vi "eFGV - Data to Execute.vi"(6 "Action":T7, 8 "Error In":errorcluster, 10 "Data to Execute":T1={"Transaction Info"={"Transaction Number"="", "Order Number"="", "Quantity"=0, "Customer"=0, "Customer Description"="", "Project"="", "Sales Order"=0, "Material"="", "Material Description"="", "Rework"=FALSE, "NCR No."="", "Ref Order No."="", "Item No."=0, "BOM Rev."=0.0}, "Product Info"={"Product Category"="", "Procedure No./Ref."="", "Test System"="", "Test System Description"="", "Working Pressure"="", "Pressure Unit"="", "Rev."="", "PSL"=""}, "Misc - Additional Refs"=[], "Misc - Sensors"=[], "Misc - Tools"=[], "Acceptance Criteria Info"={"Max Start Hold Pressure"=0.0, "Enum.Max Start Hold Pressure"=enum."%", "Permitted Hold Pressure Drop"=0.0, "Enum.Permitted Hold Pressure Drop"=enum."%", "Pressure stabilize wait time"=10.0, "Enum.Pressure stabilize wait time"=enum."minutes"}, "Execution Info"={"Auto Set Marker"=FALSE, "Auto Stop Test"=FALSE}, "Results Info"={"ListBox.Output Set"="", "Output Set Description"=""}, "Notes"=""} {"Acceptance Criteria Info"."Pressure stabilize wait time" format="%#_13g"}) -> (0 "Error Out":errorcluster, 2 "Event - Data to Execute":refnum<user-event>)   [LabVIEW 2020]
uses:
  Control/State - eFGV.ctl
  Control/Data to Execute.ctl
  Control/Transaction Info.ctl
  Control/Product Info.ctl
  Control/Acceptance Criteria Info.ctl
  Control/Execution Info.ctl
  Control/Results Info.ctl
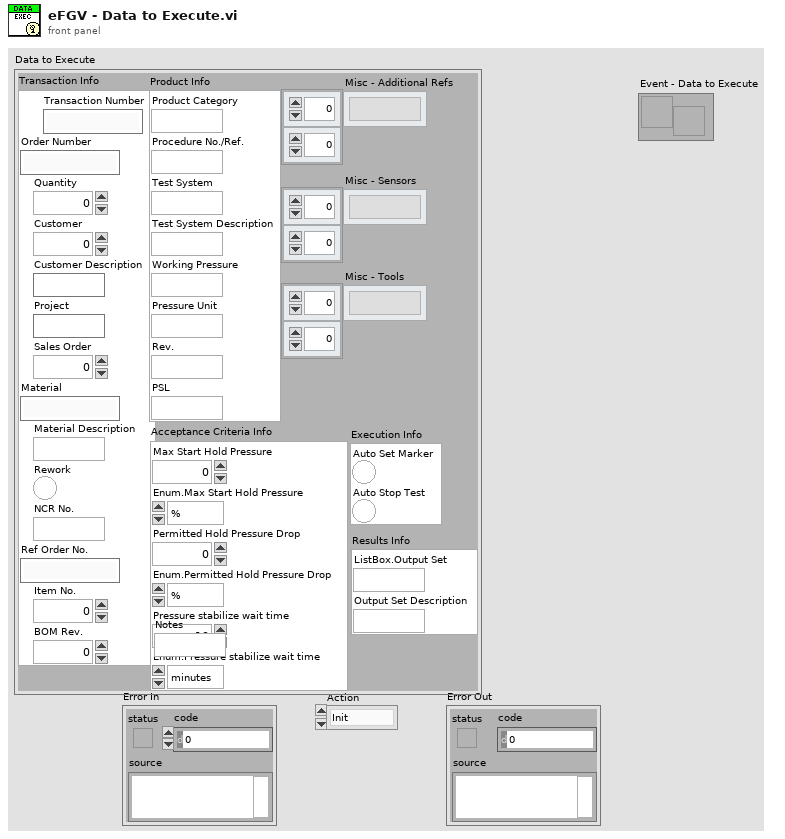
[diagram p1: front panel]
types:
  T1 = typedef "Data to Execute.ctl" = cluster{"Transaction Info":T2, "Product Info":T3, "Misc - Additional Refs":string[][], "Misc - Sensors":string[][], "Misc - Tools":string[][], "Acceptance Criteria Info":T4, "Execution Info":T5, "Results Info":T6, "Notes":string}
  T2 = typedef "Transaction Info.ctl" = cluster{"Transaction Number":string, "Order Number":string, "Quantity":u16, "Customer":u32, "Customer Description":string, "Project":string, "Sales Order":u32, "Material":string, "Material Description":string, "Rework":bool, "NCR No.":string, "Ref Order No.":string, "Item No.":u32, "BOM Rev.":dbl}
  T3 = typedef "Product Info.ctl" = cluster{"Product Category":string, "Procedure No./Ref.":string, "Test System":string, "Test System Description":string, "Working Pressure":string, "Pressure Unit":string, "Rev.":string, "PSL":string}
  T4 = typedef "Acceptance Criteria Info.ctl" = cluster{"Max Start Hold Pressure":dbl, "Enum.Max Start Hold Pressure":enum16{"%", "psi"}, "Permitted Hold Pressure Drop":dbl, "Enum.Permitted Hold Pressure Drop":enum16{"%", "psi"}, "Pressure stabilize wait time":dbl, "Enum.Pressure stabilize wait time":enum16{"seconds", "minutes"}}
  T5 = typedef "Execution Info.ctl" = cluster{"Auto Set Marker":bool, "Auto Stop Test":bool}
  T6 = typedef "Results Info.ctl" = cluster{"ListBox.Output Set":string, "Output Set Description":string}
  T7 = typedef "State - eFGV.ctl" = enum16{"Init", "Read", "Write", "Exit"}
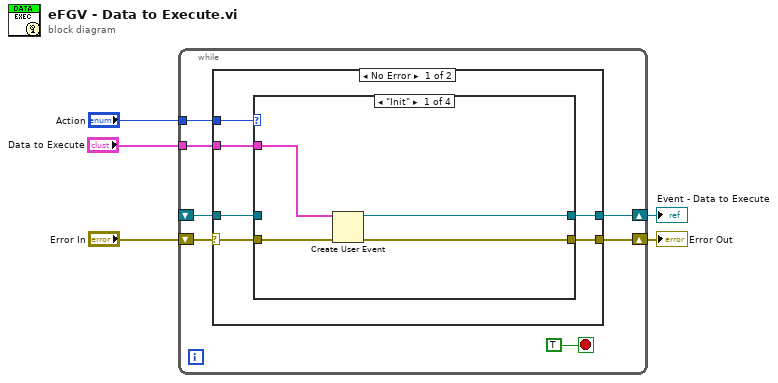
[diagram p0: block diagram]
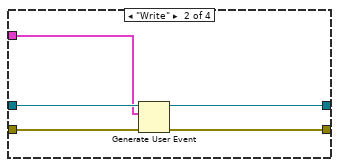
[diagram p2: hidden frame]
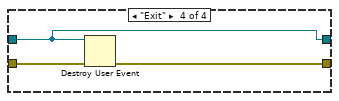
[diagram p4: hidden frame]
diagram:
  n1 = while {
    tunnel: "Action" -> [w9]
    shift-right: [w12] -> w5
    shift-left: "Error In" -> [w11]
    tunnel: "Data to Execute" -> [w8]
    shift-right: [w7] -> w1
    shift-left: _ -> [w6]
    stop <- TRUE stop-if-true
    n2 = case shown="No Error" w11 {
      selector: w11 -> [w17 w34]
      tunnel: [w18 w34] -> w12
      tunnel: w9 -> [w16 _]
      tunnel: w8 -> [w15 _]
      tunnel: [w14 w33] -> w7
      tunnel: w6 -> [w13 w33]
      frame No Error {
        n3 = case shown="\"Init\"" w16 {
          tunnel: w17 -> [w22 w27 w29 w32]
          tunnel: [w21 w26 w29 w31] -> w18
          tunnel: [w20 w25 w28 w30] -> w14
          tunnel: w15 -> [w19 w23 _ _]
          tunnel: w13 -> [_ w24 w28 w30]
          frame "Init" {
            n4 = Create User Event(user event datatype=w19, error in=w22) -> (user event=w20:refnum<user-event>, error out=w21:errorcluster)
          }
          frame "Write" {
            n5 = Generate User Event(user event=w24, event data cluster=w23, error in=w27) -> (user event out=w25:refnum<user-event>, error out=w26:errorcluster)  [unwired: 1 in]
          }
          frame "Read" {
          }
          frame "Exit" {
            n6 = Destroy User Event(user event=w30, error in=w32) -> (error out=w31:errorcluster)
          }
        }
      }
      frame Error {
      }
    }
  }
  "Error Out" <- w5
  "Event - Data to Execute" <- w1
